vi "Write Status Int.vi"(4 "error in (no error)":errorcluster, 5 "Status Value":i16 format="%04x", 6 "Status Number":u8=61, 7 "Command":T1(ring)=enum."Set Statuses") -> (0 "error out":errorcluster)   [LabVIEW 2014]
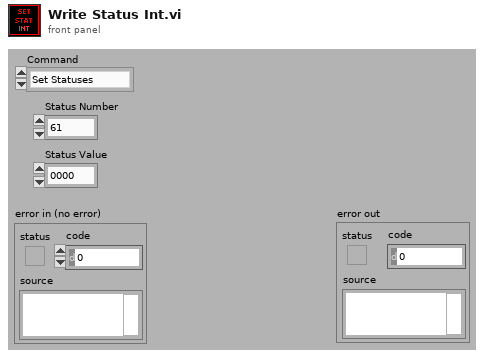
[diagram p1: front panel]
types:
  T1 = enum16{"Default", "Set Statuses", "Set Parameters", "Save Parameter"}
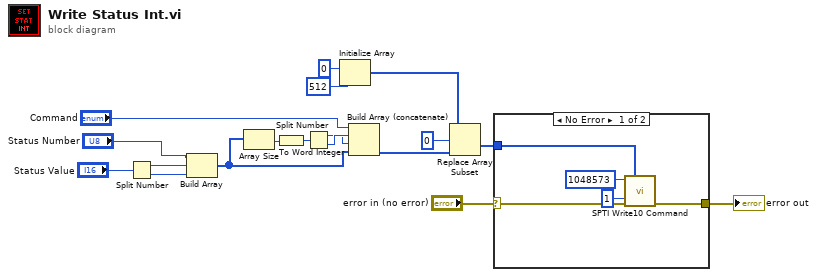
[diagram p0: block diagram]
diagram:
  n1 = Split Number(x="Status Value") -> (hi(x)=w12:u8, lo(x)=w13:u8)
  n2 = Build Array("Status Number", w12, w13) -> (w7:u8[])
  n3 = Array Size(array=w7) -> (size(s)=w1:i32)
  n4 = To Word Integer(number=w1) -> (16bit integer=w2:i16)
  n5 = Split Number(x=w2) -> (hi(x)=w3:u8, lo(x)=w4:u8)
  n6 = Initialize Array(u8 0 ("element"), 512 ("dimension size")) -> (w10:u8[])
  n7 = Build Array (concatenate)("Command", w4, w3, w7) -> (w6:u16[])
  n8 = Replace Array Subset(array=w10, new element=w6, index=0) -> (w9:u8[])
  n9 = case shown="No Error" "error in (no error)" {
    selector: "error in (no error)" -> [w20 w24]
    tunnel: [w21 w24] -> w16
    tunnel: w9 -> [w19 _]
    frame No Error {
      n10 = call "SPTI Write10 Command.vi"("Data to be Written"=w19, "error in (no error)"=w20, "Nr Blocks"=u32 1, "Start LBA"=u32 1048573) -> ("error out"=w21:errorcluster)  [unwired: 6 in, 1 out]
    }
    frame Error {
    }
  }
  "error out" <- w16
